vi "1A Helper - Sensor Status Updater.vi"(6 "Custom Error String":string, 7 "Error in":errorcluster, 8 "GPS Lock":T1, 9 "Sensor Initialized":T1, 10 "Sensor OK":T1, 11 "Sensor Connected":T1) -> ()   [LabVIEW 2011]
uses:
  2-Think/2 Typedefs/indicator LED.ctl
  2-Think/2 Globals/2 Global.vi
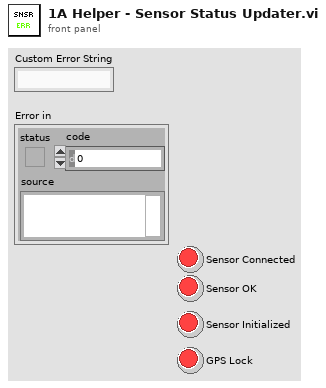
[diagram p1: front panel]
types:
  T1 = typedef "indicator LED.ctl" = bool
  T2 = typedef "generalized sensor status.ctl" = cluster{"Sensor Connected":T1, "Sensor Initialized":T1, "Sensor OK":T1, "Latest Error String":string, "GPS Lock":T1}
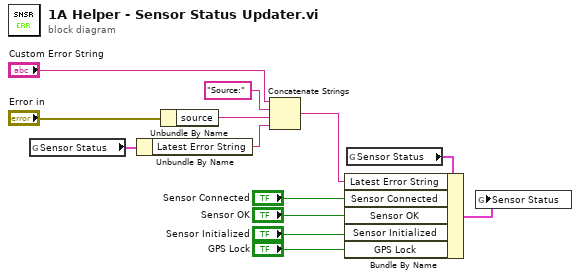
[diagram p0: block diagram]
diagram:
  n1 = global read "2 Global.vi" "Sensor Status"() -> (w4:T2)
  n2 = Unbundle By Name(w4) -> ("Latest Error String"=w3:string)
  n3 = Unbundle By Name("Error in") -> ("source"=w11:string)
  n4 = Concatenate Strings("Custom Error String", "Source:" ("string"), w11, w3) -> (w12:string)
  n5 = global read "2 Global.vi" "Sensor Status"() -> (w9:T2)
  n6 = Bundle By Name(cluster=w9, "Latest Error String"=w12, "Sensor Connected"="Sensor Connected", "Sensor OK"="Sensor OK", "Sensor Initialized"="Sensor Initialized", "GPS Lock"="GPS Lock") -> (w10:T2)
  n7 = global write "2 Global.vi" "Sensor Status"(w10) -> ()
